vi "RB2 dots to string.vi"(1 "Dot Array":T1(array[cluster])) -> (0 "dot location string":string)   [LabVIEW 2012]
doc: "This VI receives the dot location as an array of clusters and creates a single string with the data."
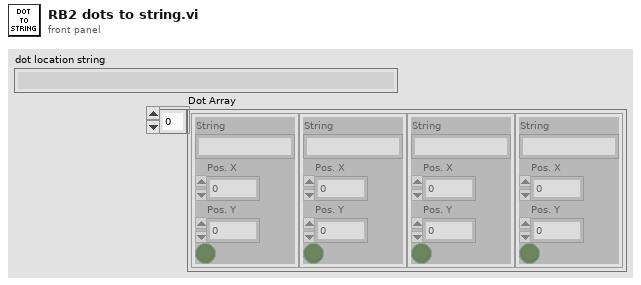
[diagram p1: front panel]
types:
  T1 = cluster{"String":string, "Pos. X":i32, "Pos. Y":i32, bool}[]
  T2 = cluster{"String":string, "Pos. X":i32, "Pos. Y":i32, bool}
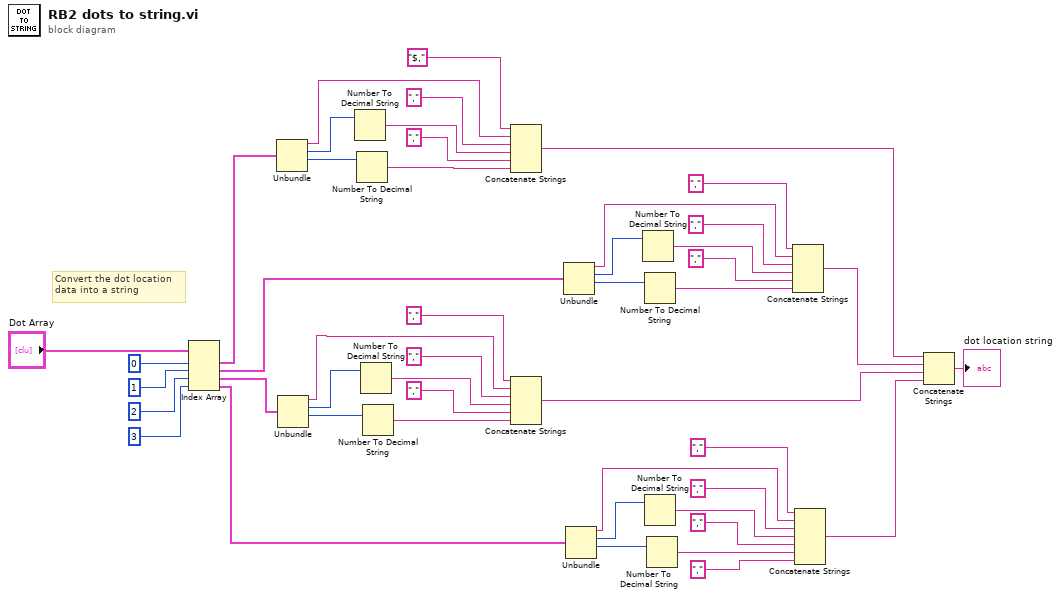
[diagram p0: block diagram]
diagram:
  # "Convert the dot location\ndata into a string"
  n1 = Index Array(array="Dot Array", index #1=0 ("index"), index #2=1 ("index"), index #3=2 ("index"), index #4=3 ("index")) -> (element #1=w43:T2, element #2=w42:T2, element #3=w41:T2, element #4=w40:T2)
  n2 = Unbundle(w43) -> ("String"=w27:string, "Pos. X"=w39:i32, "Pos. Y"=w38:i32)  [unwired: 1 out]
  n3 = Unbundle(w41) -> ("String"=w14:string, "Pos. X"=w13:i32, "Pos. Y"=w12:i32)  [unwired: 1 out]
  n4 = Number To Decimal String(number=w39) -> (decimal integer string=w37:string)  [unwired: 1 in]
  n5 = Number To Decimal String(number=w38) -> (decimal integer string=w35:string)  [unwired: 1 in]
  n6 = Number To Decimal String(number=w13) -> (decimal integer string=w22:string)  [unwired: 1 in]
  n7 = Number To Decimal String(number=w12) -> (decimal integer string=w20:string)  [unwired: 1 in]
  n8 = Concatenate Strings("$,", w27, ",", w37, ",", w35) -> (w6:string)
  n9 = Concatenate Strings(",", w14, ",", w22, ",", w20) -> (w4:string)
  n10 = Unbundle(w42) -> ("String"=w25:string, "Pos. X"=w29:i32, "Pos. Y"=w30:i32)  [unwired: 1 out]
  n11 = Unbundle(w40) -> ("String"=w10:string, "Pos. X"=w9:i32, "Pos. Y"=w8:i32)  [unwired: 1 out]
  n12 = Number To Decimal String(number=w29) -> (decimal integer string=w33:string)  [unwired: 1 in]
  n13 = Number To Decimal String(number=w30) -> (decimal integer string=w31:string)  [unwired: 1 in]
  n14 = Number To Decimal String(number=w9) -> (decimal integer string=w18:string)  [unwired: 1 in]
  n15 = Number To Decimal String(number=w8) -> (decimal integer string=w16:string)  [unwired: 1 in]
  n16 = Concatenate Strings(",", w25, ",", w33, ",", w31) -> (w5:string)
  n17 = Concatenate Strings(",", w10, ",", w18, ",", w16, ",") -> (w3:string)
  n18 = Concatenate Strings(w6, w5, w4, w3) -> (→"dot location string":string)
